vi "Create.vi"(5 "TestCaseMock In":refnum<class "TestCaseMock.lvclass">, 8 "error in (no error)":errorcluster) -> (0 "error out":errorcluster, 3 "TestCaseMock":refnum<class "TestCaseMock.lvclass">)   [LabVIEW 2017, in "TestSuite.Tests.lvlib" / "Support.lvlib" / "TestCaseMock.lvclass"]
uses:
  TestCaseMock.lvclass
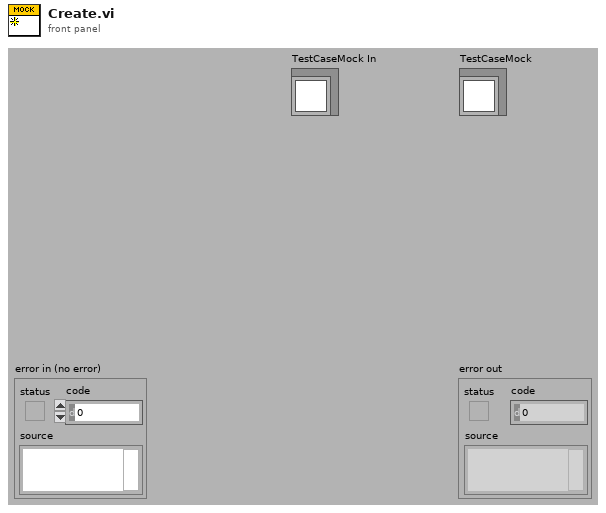
[diagram p1: front panel]
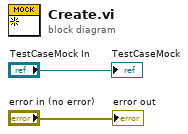
[diagram p0: block diagram]
diagram:
  "error out" <- "error in (no error)"
  "TestCaseMock" <- "TestCaseMock In"
